vi "SUB_COM9_INIT_Jerry.vi"(3 "baud rate":u32=9600) -> (0 "error out":errorcluster, 1 "VISA resource name out":refnum<visa-resource-name>)   [LabVIEW 2011]
uses:
  <vilib>/Instr/_visa.llb/VISA Configure Serial Port (Instr).vi
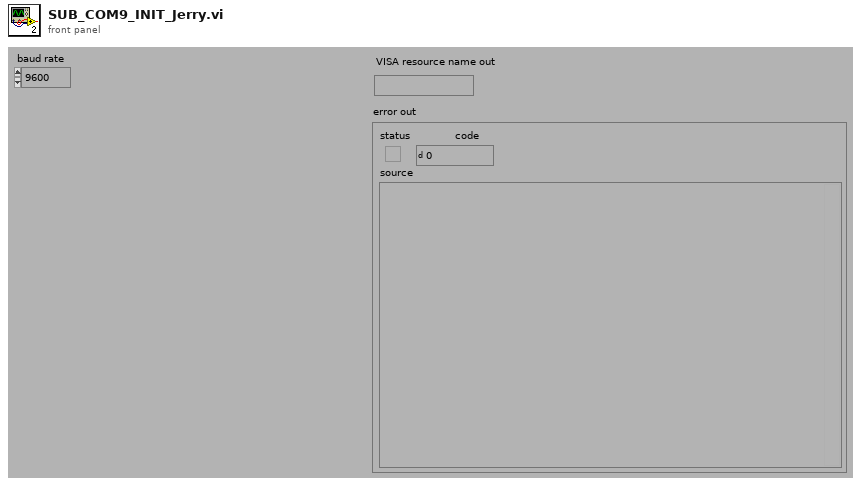
[diagram p1: front panel]
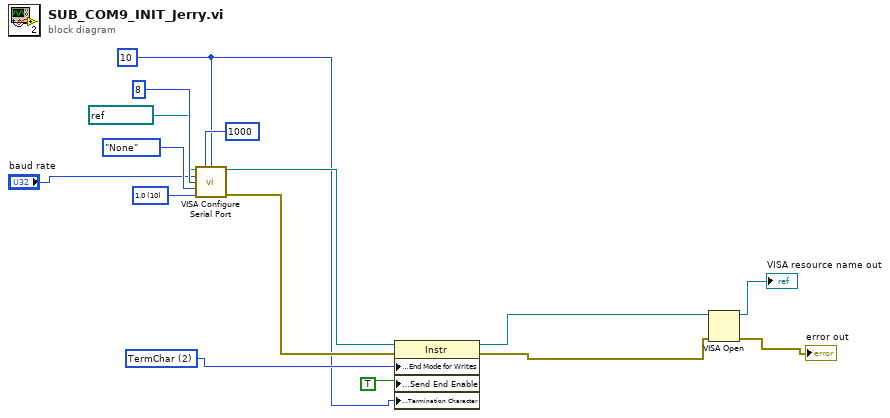
[diagram p0: block diagram]
diagram:
  w6 = u16 2 items=["None", "LastBit", "TermChar", "Break"] ("Serial Settings:Serial End Mode for Writes")
  w1 = u8 10 ("termination char\n(0xA = '\\n' = LF)")
  w14 = u16 10 items=["1.0"=10, "1.5"=15, "2.0"=20] ("stop bits (10: 1 bit)")
  n1 = call-poly "VISA Configure Serial Port"("VISA resource name"=refnum<visa-resource-name> "COM9", "timeout (10sec)"=u32 1000, "termination char\n(0xA = '\\n' = LF)"=w1, "baud rate (9600)"="baud rate", "data bits (8)"=u16 8, "parity (0:none)"=enum16{"None", "Odd", "Even", "Mark", "Space"}."None", "stop bits (10: 1 bit)"=w14) -> ("VISA resource name out"=w5:refnum<visa-resource-name>, "error out"=w2:errorcluster)  [unwired: 7 in]
  n2 = property class="Instr"(reference=w5, error in=w2, "Serial Settings:End Mode for Writes"=w6, "Message Based Settings:Send End Enable"=TRUE ("End write with termination character?"), "Message Based Settings:Termination Character"=w1) -> (reference out=w4:refnum<visa-resource-name>, error out=w3:errorcluster)
  n3 = VISA Open(error in (no error)=w3, VISA resource name=w4) -> (VISA resource name=→"VISA resource name out":refnum<visa-resource-name>, error out=→"error out":errorcluster)  [unwired: 3 in]
